vi "FP forebrain ACT.vi"(2 "error in":errorcluster, 3 "local Steering\nangle":dbl=-135.0 format="%#_13g", 4 "Behaviors in":T1) -> (0 "error out":errorcluster, 1 "Forebrain ACT":dbl[](array[numeric]))   [LabVIEW 2014]
panel:
  out "Forebrain ACT Graph":cluster{dbl, dbl, dbl[]}(graph)
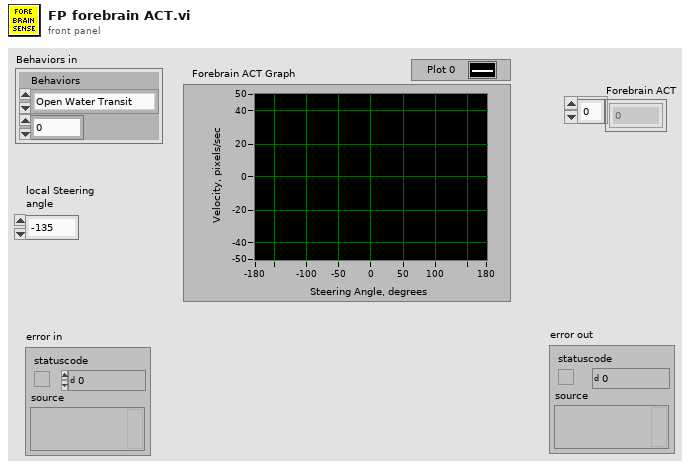
[diagram p1: front panel]
types:
  T1 = cluster{"Behaviors":enum16{"Open Water Transit", "P-Wall Follow", "S-Wall Follow", "Dock"}, dbl}
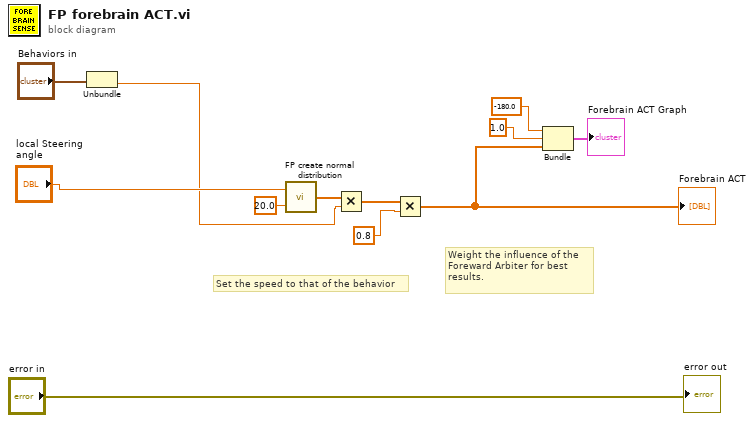
[diagram p0: block diagram]
diagram:
  # "Weight the influence of the\nForeward Arbiter for best\nresults."
  # "Set the speed to that of the behavior"
  n1 = Unbundle("Behaviors in") -> (w4:dbl)  [unwired: 1 out]
  n2 = call "FP create normal distribution.vi"("std (Normal)"=20.0, "mean"="local Steering\nangle") -> ("ACT array"=w10:dbl[])
  n3 = Multiply(x=w10, y=w4) -> (x*y=w3:dbl[])
  n4 = Multiply(x=w3, y=0.8 ("Arbiter weight")) -> (x*y=w2:dbl[])
  "Forebrain ACT" <- w2
  n5 = Bundle(-180.0, 1.0, w2) -> (→"Forebrain ACT Graph":cluster{dbl, dbl, dbl[]})  [unwired: 1 in]
  "error out" <- "error in"
